vi "Set Visible From Object.vi"(8 "error in (no error)":errorcluster, 11 "Object in":refnum<class "Object.lvclass">) -> (0 "error out":errorcluster, 3 "Object out":refnum<class "Object.lvclass">)   [LabVIEW 2021, in "Object.lvclass"]
uses:
  Object.lvclass
  Object.lvclass/Object.ctl
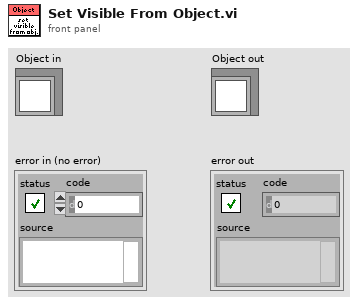
[diagram p1: front panel]
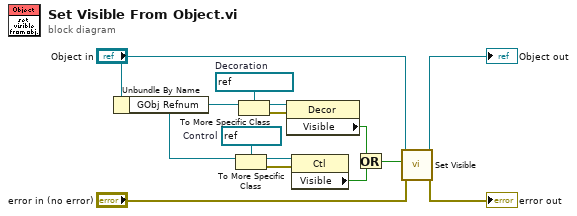
[diagram p0: block diagram]
diagram:
  w10 = refnum<vi> refnum  # Control
  w13 = refnum<vi> refnum  # Decoration
  n1 = Unbundle By Name("Object in") -> ("GObj Refnum"=w8:refnum<vi>)
  n2 = To More Specific Class(target class=w10, reference=w8) -> (specific class reference=w9:refnum<vi>, error out=w11:errorcluster)  [unwired: 1 in]
  n3 = To More Specific Class(target class=w13, reference=w8) -> (specific class reference=w14:refnum<vi>, error out=w12:errorcluster)  [unwired: 1 in]
  n4 = property class="Decor"(reference=w14, error in=w12) -> ("Visible"=w7:bool)  [unwired: 2 out]
  n5 = property class="Ctl"(reference=w9, error in=w11) -> ("Visible"=w6:bool)  [unwired: 2 out]
  n6 = Or(x=w7, y=w6) -> (x .or. y?=w5:bool)
  n7 = call-dynamic "Set Visible.vi"("error in (no error)"="error in (no error)", "Show? [T]"=w5, "MMI Scaling in"="Object in") -> ("error out"=→"error out":errorcluster, "MMI Scaling out"=→"Object out":refnum<class "Object.lvclass">)  [unwired: 7 in]
